vi "PID_Separate(subvi)_v.vi"(10 "setpoint":dbl[](array[numeric])=[0.0, 0.0, 0.0, 0.0] format="%.2f", 11 "PID gains":T1(array[cluster])=[{"proportional gain (Kc)"=3.37, "integral time (Ti, min)"=0.004, "derivative time (Td, min)"=0.0}, {"proportional gain (Kc)"=3.37, "integral time (Ti, min)"=0.004, "derivative time (Td, min)"=0.0}, {"proportional gain (Kc)"=3.37, "integral time (Ti, min)"=0.004, "derivative time (Td, min)"=0.0}, {"proportional gain (Kc)"=3.37, "integral time (Ti, min)"=0.004, "derivative time (Td, min)"=0.0}] {"derivative time (Td, min)" format="%.3f"; "integral time (Ti, min)" format="%.3f"; "proportional gain (Kc)" format="%.3f"}) -> ()   [LabVIEW 2018]
uses:
  <vilib>/addons/control/pid/pid.llb/PID (DBL Array).vi
  <vilib>/addons/control/pid/NI_PID_pid.lvlib
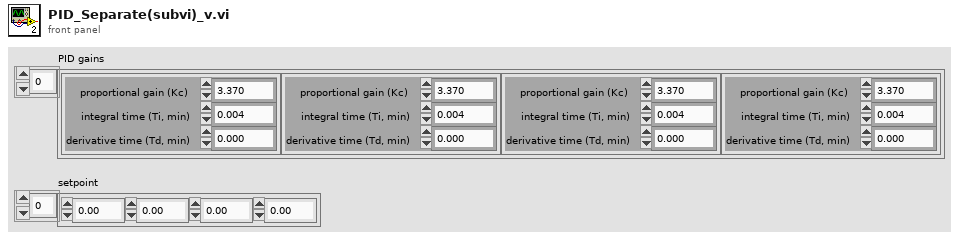
[diagram p1: front panel]
types:
  T1 = cluster{"proportional gain (Kc)":dbl, "integral time (Ti, min)":dbl, "derivative time (Td, min)":dbl}[]
  T2 = cluster{bool, "Tick Count(uSec)":u32, "Counter Value":i32[], "x-y":i32[]}
  T3 = cluster{"Position":i32[], "Velocity RPM":dbl[], "Velocity RPS":dbl[], "Radians/s":dbl[]}
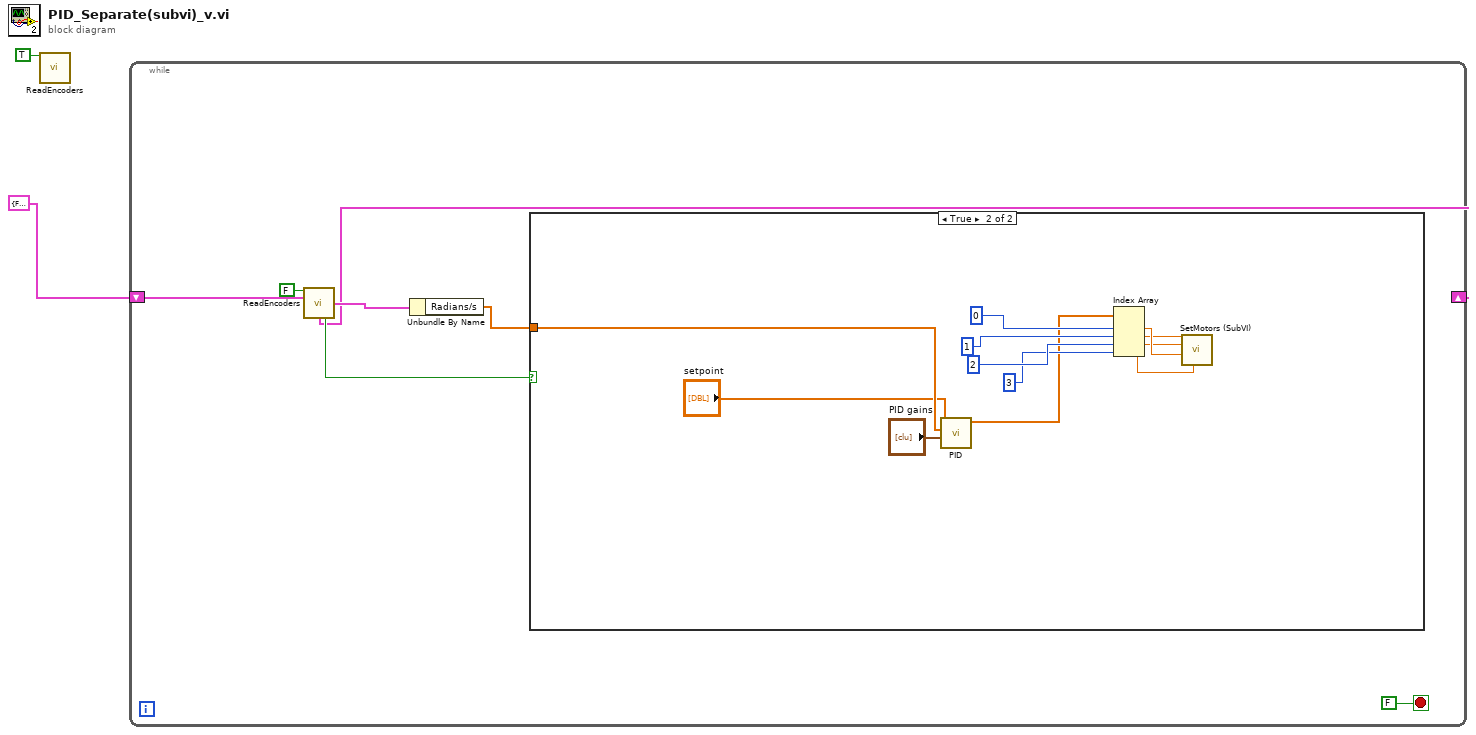
[diagram p0: block diagram]
diagram:
  n1 = call "ReadEncoders.vi"("Reset Encoders"=TRUE) -> ()  [unwired: 10 in, 5 out]
  n2 = while {
    shift-right: [w4] -> _
    shift-left: T2 {FALSE, "Tick Count(uSec)"=0, "Counter Value"=[0, 0, 0, 0], "x-y"=[0, 0, 0, 0]} ("Cluster in") -> [w5]
    stop <- FALSE stop-if-true
    n3 = call "ReadEncoders.vi"("Reset Encoders"=FALSE, "Cluster in"=w5) -> ("output cluster"=w9:T3, "Cluster Out"=w4:T2, "Updated"=w8:bool)  [unwired: 9 in, 2 out]
    n4 = Unbundle By Name(w9) -> ("Radians/s"=w6:dbl[])
    n5 = case shown="True" w8 {
      tunnel: w6 -> [_ w21]
      frame False {
      }
      frame True {
        n6 = call-poly <vilib>:"PID.vi"("PID gains"="PID gains", "process variable"=w21, "setpoint"="setpoint") -> ("output"=w15:dbl[])  [unwired: 7 in, 1 out]
        n7 = Index Array(array=w15, index #1=0 ("index"), index #2=1 ("index"), index #3=2 ("index"), index #4=3 ("index")) -> (element #1=w13:dbl, element #2=w12:dbl, element #3=w11:dbl, element #4=w10:dbl)
        n8 = call "SetMotors (SubVI).vi"("Oikea"=w10, "Etu"=w13, "Vasen"=w11, "Taka"=w12) -> ()  [unwired: 8 in]
      }
    }
  }
